vi "CheckSet STOP.vi"(7 "stop value":bool, 9 "error in (no error)":errorcluster) -> (8 "Boolean":bool, 10 "error out":errorcluster)   [LabVIEW 2010, in "GlobalStop(dev).lvlib"]
uses:
  GlobalStop(dev).lvlib
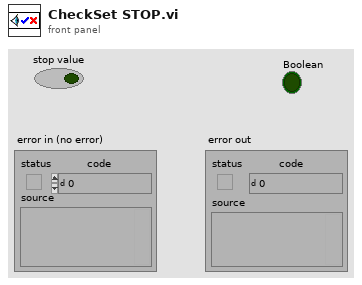
[diagram p1: front panel]
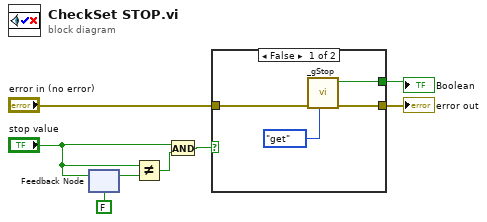
[diagram p0: block diagram]
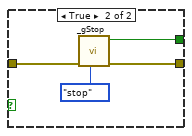
[diagram p2: hidden frame]
diagram:
  n1 = feedback-in #1("stop value") -> ()
  n2 = feedback #1(FALSE ("stop value")) -> (w4:bool)
  n3 = Not Equal?(x="stop value", y=w4) -> (x != y?=w3:bool)
  n4 = And(x="stop value", y=w3) -> (x .and. y?=w2:bool)
  n5 = case shown="False" w2 {
    tunnel: "error in (no error)" -> [w10 w16]
    tunnel: [w9 w15] -> w7
    tunnel: [w12 w14] -> w6
    frame False {
      n6 = call "_gStop.vi"("op"=enum16{"reset", "get", "stop"}."get", "error in (no error)"=w10) -> ("error out"=w9:errorcluster, "Boolean"=w12:bool)  [unwired: 8 in]
    }
    frame True {
      n7 = call "_gStop.vi"("op"=enum16{"reset", "get", "stop"}."stop", "error in (no error)"=w16) -> ("error out"=w15:errorcluster, "Boolean"=w14:bool)  [unwired: 8 in]
    }
  }
  "error out" <- w7
  "Boolean" <- w6
